vi "Rec Delete.vi"(4 "error in (no error)":errorcluster, 7 "recordset reference":T3) -> (0 "error out":errorcluster, 2 "data":T1, 3 "object name":string)   [LabVIEW 2017, in "NI_Database_API.lvlib"]
doc: "Deletes a <B>Recordset</B> object created with the <B>Rec New</B> VI and returns the contents of the object."
uses:
  <vilib>/addons/database/NI_Database_API.lvlib
  <vilib>/addons/database/Recordset.llb/Rec ObjectReference.ctl
  <vilib>/addons/database/Recordset.llb/Rec DataMembers.ctl
  <vilib>/addons/database/Connection.llb/Conn ObjectReference.ctl
  <vilib>/Utility/_goopsup.llb/GOOP Object Repository Method.ctl
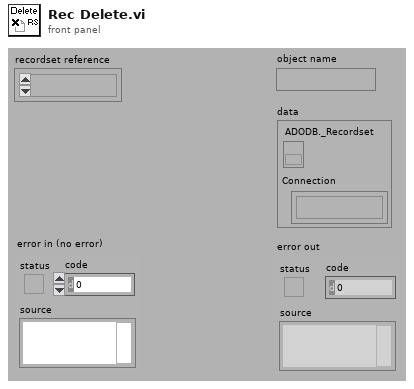
[diagram p1: front panel]
types:
  T1 = typedef "NI_Database_API.lvlib/Rec DataMembers.ctl" = cluster{"ADODB._Recordset":refnum<k7>, "Connection":T2}
  T2 = typedef "NI_Database_API.lvlib/Conn ObjectReference.ctl" = refnum<k1>
  T3 = typedef "NI_Database_API.lvlib/Rec ObjectReference.ctl" = refnum<k1>
  T4 = typedef "GOOP Object Repository Method.ctl" = enum16{"Create", "GetCopy", "GetModify", "Set", "Destroy", "Create Static", "Get All Refs", "Reset", "Get Statistics"}
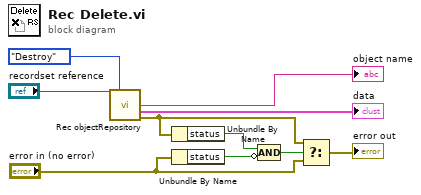
[diagram p0: block diagram]
diagram:
  n1 = call <vilib>:"Rec objectRepository.vi"("recordset reference"="recordset reference", "method"=GOOP_Object_Repository_Method."Destroy") -> ("name out"=→"object name":string, "classDataOut"=→"data":T1, "error out"=w6:errorcluster)  [unwired: 7 in, 4 out]
  n2 = Unbundle By Name(w6) -> ("status"=w3:bool)
  n3 = Unbundle By Name("error in (no error)") -> ("status"=w2:bool)
  n4 = Compound Arithmetic op=AND(w3, invert w2) -> (w1:bool)
  n5 = Select(t=w6, s=w1, f="error in (no error)") -> (s? t:f=→"error out":errorcluster)
